vi "Update_Moving.vi"(8 "error in (no error)":errorcluster, 9 "Moving?":bool, 10 "PV-URL":string, 11 "CS++Motor in":refnum<class "CS++Motor.lvclass">) -> (0 "error out":errorcluster, 3 "CS++Motor out":refnum<class "CS++Motor.lvclass">)   [LabVIEW 2015, in "CS++Motor.lvlib" / "CS++Motor.lvclass"]
doc: "This VI is executed via the corresponding Monitor Actor and delivers the information wether an axis is moving or not."
uses:
  CS++Motor.lvclass
  CS++Motor.lvclass/CS++Motor.ctl
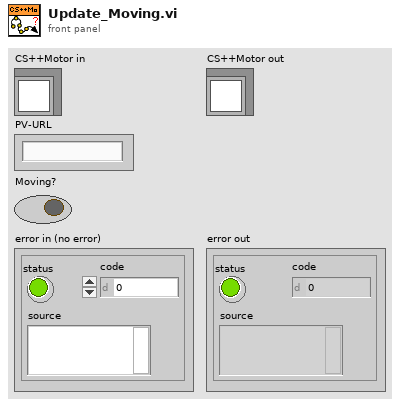
[diagram p1: front panel]
types:
  T1 = cluster{"Command":string, "AxisNumber":u8, "Data":variant}
  T2 = cluster{"Update-Msg Name":string, "Update-Msg URLs":string[]}[]
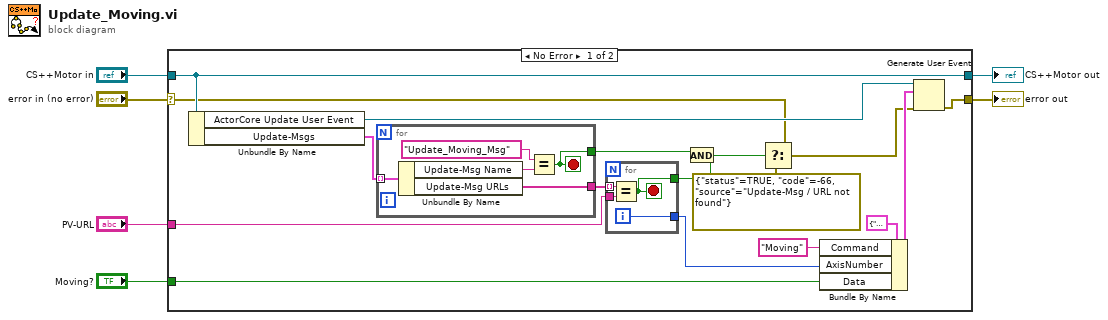
[diagram p0: block diagram]
diagram:
  n1 = case shown="No Error" "error in (no error)" {
    selector: "error in (no error)" -> [w9 w34]
    tunnel: [w21 w34] -> w5
    tunnel: [w18 w33] -> w3
    tunnel: "CS++Motor in" -> [w18 w33]
    tunnel: "Moving?" -> [w19 _]
    tunnel: "PV-URL" -> [w11 _]
    frame No Error {
      n2 = Unbundle By Name(w18) -> ("ActorCore Update User Event"=w17:refnum<user-event>, "Update-Msgs"=w10:T2)
      n3 = for {
        tunnel: w10 -> [w32] mode=indexing
        tunnel: [w29] -> w16
        tunnel: [w28] -> w15
        stop <- w28 stop-if-true
        n4 = Unbundle By Name(w32) -> ("Update-Msg Name"=w31:string, "Update-Msg URLs"=w29:string[])
        n5 = Equal?(x="Update_Moving_Msg", y=w31) -> (x = y?=w28:bool)
      }
      n6 = for {
        tunnel: w16 -> [w27] mode=indexing
        tunnel: w11 -> [w26]
        tunnel: [w25] -> w14
        tunnel: [w24] -> w7
        i -> [w24]
        stop <- w25 stop-if-true
        n7 = Equal?(x=w27, y=w26) -> (x = y?=w25:bool)
      }
      n8 = And(x=w15, y=w14) -> (x .and. y?=w13:bool)
      n9 = Select(t=w9, s=w13, f=errorcluster {"status"=TRUE, "code"=-66, "source"="Update-Msg / URL not found"}) -> (s? t:f=w8:errorcluster)
      n10 = Bundle By Name(cluster=T1 {"Command"="", "AxisNumber"=0, "Data"=variant} ("event data"), "Command"="Moving", "AxisNumber"=w7, "Data"=w19) -> (w22:T1)
      n11 = Generate User Event(user event=w17, event data cluster=w22, error in=w8) -> (error out=w21:errorcluster)  [unwired: 1 in, 1 out]
    }
    frame Error {
    }
  }
  "error out" <- w5
  "CS++Motor out" <- w3
